vi "PressureTransducer.vi"(1 "FieldPoint IO Point In":refnum<k21>) -> (0 "psi":dbl)   [LabVIEW 2012]
uses:
  <vilib>/FieldPoint/Polymorphic Read.llb/FP Read (Float -IO).vi
panel:
  in  "?":bool
  # "Pressure Measurement (Transducer)"
  # "(Excitation: 9 to 30 VDC )"
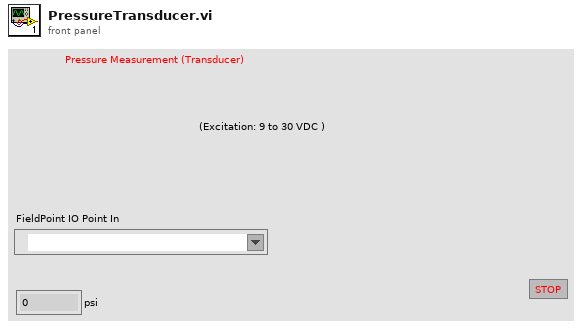
[diagram p1: front panel]
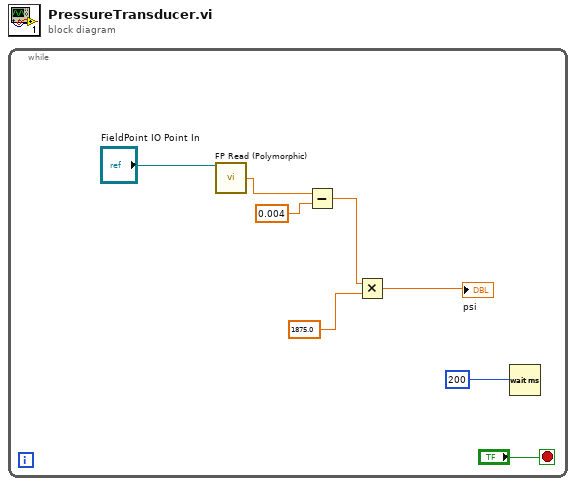
[diagram p0: block diagram]
diagram:
  n1 = while {
    stop <- "?" stop-if-true
    n2 = call-poly <vilib>:"FP Read (Polymorphic).vi"("FieldPoint IO Point In"="FieldPoint IO Point In") -> ("value"=w4:dbl)  [unwired: 11 in, 3 out]
    n3 = Subtract(x=w4, y=0.004) -> (x-y=w2:dbl)
    n4 = Multiply(x=w2, y=1875.0) -> (x*y=→"psi":dbl)
    n5 = Wait (ms)(milliseconds to wait=u32 200) -> ()  [unwired: 1 out]
  }
